vi "Transmitter.vi"() -> ()   [LabVIEW 2013]
uses:
  <vilib>/sound2/lvsound2.llb/Sound File Info (path).vi
  <vilib>/sound2/lvsound2.llb/Sound File Read Open.vi
  <vilib>/Analysis/2dsp.llb/Rational Resample (single channel, DBL).vi
  <instrlib>/niUSRP/niUSRP Write Tx Data (CDB).vi
  <vilib>/sound2/lvsound2.llb/Sound File Read (DBL).vi
  <vilib>/Analysis/NI_AALPro.lvlib
panel:
  out "Constellatiom":cluster{dbl[], dbl[]}(graph)
  in  "stop":bool
  out "error out":errorcluster
  in  "FM deviation":dbl=75000.0 format="%#_6f"
  out "output waveform":waveform(dbl)(graph)
  in  "active antenna":string="TX1"
  out "coerced gain":dbl format="%#_6p"
  out "coerced carrier frequency":dbl=2400000000.0 format="%#_6p"
  out "coerced IQ rate":dbl=200000.0 format="%#_6p"
  in  "IP":refnum<k15>="192.168.10.2"
  in  "path":path=path "E:/TianyangChen/ComProject_I/LoveUSRP/International.wav"
  in  "number of samples":i32=11025
  in  "gain":dbl format="%#_6f"
  in  "carrier frequency":dbl=2400000000.0 format="%#_6p"
  in  "IQ rate":dbl=200000.0 format="%#_6p"
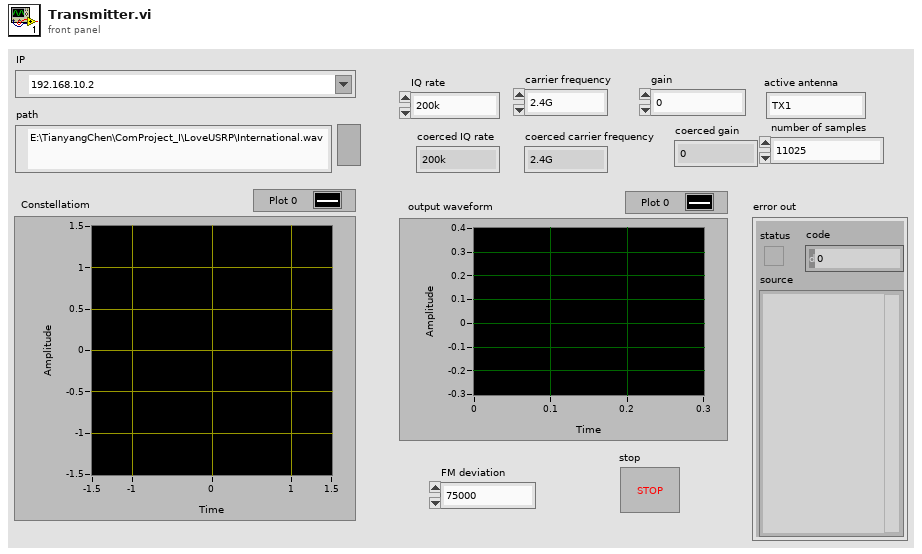
[diagram p1: front panel]
types:
  T1 = typedef "Sound Data Format.ctl" = cluster{"sample rate (S/s)":dbl, "number of channels":i32, "bits per sample":i32}
  T2 = typedef "Sound File Refnum.ctl" = refnum<file>
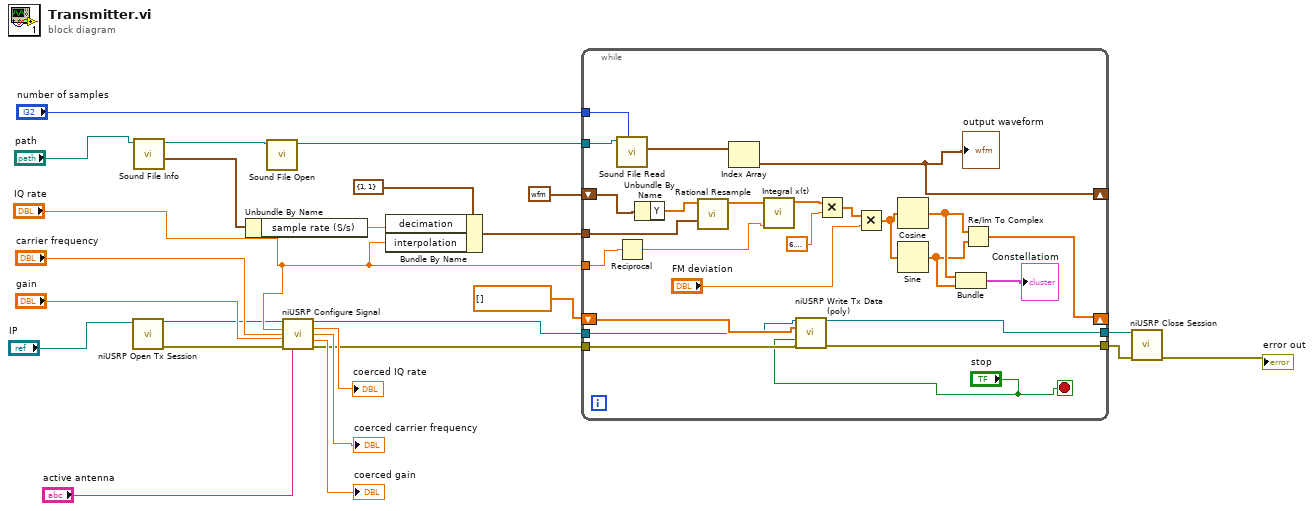
[diagram p0: block diagram]
diagram:
  n1 = call <instrlib>:"niUSRP Open Tx Session.vi"("device names"="IP") -> ("session handle out"=w1:refnum<k15>, "error out"=w21:errorcluster)  [unwired: 13 in]
  n2 = call-poly <vilib>:"Sound File Info.vi"("path"="path") -> ("sound format"=w15:T1, "path out"=w25:path)  [unwired: 7 in, 2 out]
  n3 = Unbundle By Name(w15) -> ("sample rate (S/s)"=w14:dbl)
  n4 = call-poly <vilib>:"Sound File Open.vi"("path"=w25) -> ("sound file refnum"=w24:T2)  [unwired: 9 in, 1 out]
  n5 = call <instrlib>:"niUSRP Configure Signal.vi"("session handle"=w1, "IQ rate"="IQ rate", "carrier frequency"="carrier frequency", "gain"="gain", "error in (no error)"=w21, "active antenna"="active antenna") -> ("session handle out"=w13:refnum<k15>, "coerced IQ rate"=→"coerced IQ rate":dbl, "coerced carrier frequency"=→"coerced carrier frequency":dbl, "coerced gain"=→"coerced gain":dbl, "error out"=w10:errorcluster)  [unwired: 5 in]
  n6 = Bundle By Name(cluster=cluster{"interpolation":i32, "decimation":i32} {"interpolation"=1, "decimation"=1} ("input cluster"), "decimation"=w14, "interpolation"="IQ rate") -> (w6:cluster{"interpolation":i32, "decimation":i32})
  n7 = while {
    tunnel: w24 -> [w50]
    tunnel: "number of samples" -> [w49]
    shift-right: [w46] -> _
    shift-left: waveform(dbl) {"t0"=timestamp(0 s since 1904-01-01), "dt"=1.0, "Y"=[]} ("waveform") -> [w47]
    shift-right: [w35] -> _
    shift-left: cdb[] [] ("data") -> [w34]
    tunnel: w13 -> [w33]
    tunnel: [w32] -> w12
    tunnel: [w31] -> w11
    tunnel: w10 -> [w30]
    tunnel: w6 -> [w29]
    tunnel: "IQ rate" -> [w26]
    stop <- "stop" stop-if-true
    n8 = call-poly <vilib>:"Sound File Read.vi"("number of samples/ch (-1: all)"=w49, "sound file refnum"=w50) -> ("data"=w48:waveform(dbl)[])  [unwired: 5 in, 4 out]
    n9 = Reciprocal(x=w26) -> (1/x=w43:dbl)
    n10 = Unbundle By Name(w47) -> ("Y"=w45:dbl[])
    n11 = call-poly <vilib>:"Rational Resample.vi"("resample factor"=w29, "X"=w45) -> ("Y"=w44:dbl[])  [unwired: 7 in, 2 out]
    n12 = Index Array(array=w48) -> (element=w46:waveform(dbl))  [unwired: 1 in]
    "output waveform" <- w46
    n13 = call <vilib>:"Integral x(t).vi"("dt"=w43, "X"=w44) -> ("Integral X"=w42:dbl[])  [unwired: 8 in, 1 out]
    n14 = call-poly <instrlib>:"niUSRP Write Tx Data (poly).vi"("session handle"=w33, "data"=w34, "end of data?"="stop", "error in (no error)"=w30) -> ("session handle out"=w32:refnum<k15>, "error out"=w31:errorcluster)  [unwired: 10 in]
    n15 = Multiply(x=w42, y=6.283185307179586) -> (x*y=w41:dbl[])
    n16 = Multiply(x=w41, y="FM deviation") -> (x*y=w38:dbl[])
    n17 = Cosine(x=w38) -> (cos(x)=w37:dbl[])
    n18 = Sine(x=w38) -> (sin(x)=w36:dbl[])
    n19 = Bundle(w37, w36) -> (→"Constellatiom":cluster{dbl[], dbl[]})  [unwired: 1 in]
    n20 = Re/Im To Complex(1:w36, 2:w37) -> (0:w35:cdb[])
  }
  n21 = call <instrlib>:"niUSRP Close Session.vi"("session handle"=w12, "error in (no error)"=w11) -> ("error out"=→"error out":errorcluster)  [unwired: 13 in]
